vi "ACT_6_Task2_825005609.vi"() -> ()   [LabVIEW 2016]
panel:
  out "String":string
  in  "Switch":bool
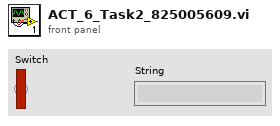
[diagram p1: front panel]
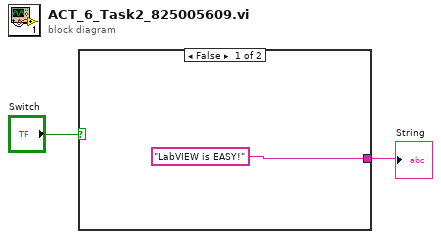
[diagram p0: block diagram]
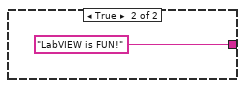
[diagram p2: hidden frame]
diagram:
  n1 = case shown="False" "Switch" {
    tunnel: ["LabVIEW is EASY!" ("String") "LabVIEW is FUN!" ("String")] -> w1
    frame False {
    }
    frame True {
    }
  }
  "String" <- w1
